vi "create_class2_ref.vi"() -> (3 "Class 2.lvclass":refnum<class "Class 2.lvclass">)   [LabVIEW 2023]
uses:
  class2/Class 2.lvclass
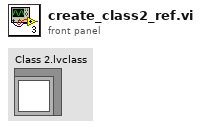
[diagram p1: front panel]
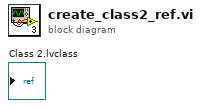
[diagram p0: block diagram]
diagram:
